vi "Vision.vi"() -> (3 "Done?":bool=TRUE)   [LabVIEW 2019]
uses:
  <vilib>/addons/control/pid/autopid.llb/PID autotuning parameters (adv).ctl
  <vilib>/Rock Robotics/WPI/Utilities/WPI_GetSetVariantRefNum.vi
  <vilib>/Rock Robotics/Network Tables/NT Write Boolean Array.vi
  <vilib>/Rock Robotics/Network Tables/NT Write Numeric Array.vi
  <vilib>/Rock Robotics/Network Tables/NT Read Boolean.vi
  <vilib>/Rock Robotics/Network Tables/NT Read Number.vi
  <vilib>/Rock Robotics/Network Tables/NT Write Boolean.vi
  <vilib>/addons/control/pid/NI_PID_autopid.lvlib
panel:
  out "tuning completed?":bool
  out "tuned PID gains":T1={"proportional gain (Kc)"=1.0, "integral time (Ti, min)"=0.01, "derivative time (Td, min)"=0.0} {"derivative time (Td, min)" format="%#.6g"; "integral time (Ti, min)" format="%#.6g"; "proportional gain (Kc)" format="%#.6g"}
  out "x/y":dbl
  in  "PID gains":T1={"proportional gain (Kc)"=0.07, "integral time (Ti, min)"=0.0033999999999999994, "derivative time (Td, min)"=0.05} {"derivative time (Td, min)" format="%.6f"; "integral time (Ti, min)" format="%.6f"; "proportional gain (Kc)" format="%.6f"}
  in  "On":bool
  out "Yaw":dbl
  out "Sample Slider 0":dbl(slide) scale=0.0..5.0
  out "Sample Boolean 1":bool
  out "Sample Boolean 0":bool
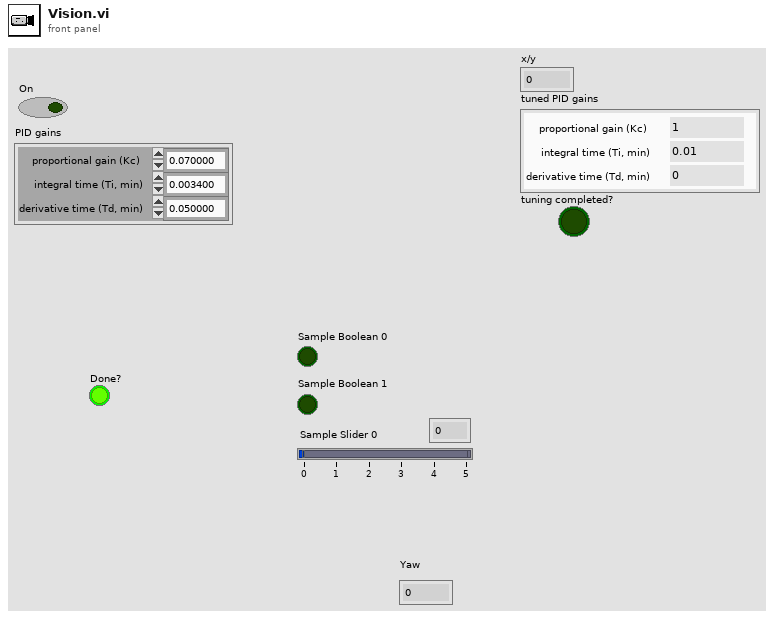
[diagram p1: front panel]
types:
  T1 = cluster{"proportional gain (Kc)":dbl, "integral time (Ti, min)":dbl, "derivative time (Td, min)":dbl}
  T2 = typedef "NI_PID_autopid.lvlib/PID autotuning parameters (adv).ctl" = cluster{"technique":u16, "type of controller":u16, "control specification":u16, "amplitude":dbl}
  T3 = typedef "WPI_EncoderDevRef.ctl" = cluster{"DevStatus":errorcluster, "EncoderIndex":T4, "CounterIndex":T5, "DistancePerCount":dbl, "Decoding Type":T6}
  T4 = typedef "FPGA_EncoderIdx.ctl" = enum8{"Enc 0", "Enc 1", "Enc 2", "Enc 3", "Enc 4", "Enc 5", "Enc 6", "Enc 7", "Invalid"}
  T5 = typedef "FPGA_CounterCtrSystemIndex.ctl" = enum8{"Ctr 0", "Ctr 1", "Ctr 2", "Ctr 3", "Ctr 4", "Ctr 5", "Ctr 6", "Ctr 7", "Invalid"}
  T6 = typedef "WPI_EncoderType.ctl" = enum16{"1x", "2x", "4x"}
  T7 = typedef "WPI_MotorControlDeviceRef.ctl" = cluster{"DeviceStatus":errorcluster, "Type":T8, "PWM":cluster{"PWM Channel":T9, "DeadBand":T10}, "CAN":cluster{"Device Number":u8, "SetOutput VI Ref":variant, "GetOutput VI Ref":variant, "Enable VI Ref":variant, "Disable VI Ref":variant, "Data":variant}, "Invert":bool, "DIO PWM":cluster{"PWM \"Enable\" Channel":T9, "DIOChannel":T11, "PWM Rate":dbl}}
  T8 = typedef "WPI_MotorControlType.ctl" = enum16{"PWM", "CAN", "DIO PWM"}
  T9 = typedef "FPGA_DIOPWMChannel.ctl" = enum8{"PWM 0", "PWM 1", "PWM 2", "PWM 3", "PWM 4", "PWM 5", "PWM 6", "PWM 7", "PWM 8", "PWM 9", "PWM MXP 0", "PWM MXP 1", "PWM MXP 2", "PWM MXP 3", "PWM MXP 4", "PWM MXP 5", "PWM MXP 6", "PWM MXP 7", "PWM MXP 8", "PWM MXP 9", "Invalid"}
  T10 = typedef "WPI_PWMDeadband.ctl" = cluster{"Name":string, "maxPositivePwm":i32, "minPositivePwm":i32, "centerPwm":i32, "maxNegativePwm":i32, "minNegativePwm":i32, "angularRange":u16}
  T11 = typedef "FPGA_DIOChannel.ctl" = enum8{"DIO 0", "DIO 1", "DIO 2", "DIO 3", "DIO 4", "DIO 5", "DIO 6", "DIO 7", "DIO 8", "DIO 9", "DIO MXP 0", "DIO MXP 1", "DIO MXP 2", "DIO MXP 3", "DIO MXP 4", "DIO MXP 5", "DIO MXP 6", "DIO MXP 7", "DIO MXP 8", "DIO MXP 9", "DIO MXP 10", "DIO MXP 11", "DIO MXP 12", "DIO MXP 13", "DIO MXP 14", "DIO MXP 15", "SPI Port CS1", "SPI Port CS2", "SPI Port CS3", "SPI Port MISO", "SPI Port MOSI", "Invalid"}
  T12 = typedef "WPI_JoystickDevRef.ctl" = cluster{"Device":T13}
  T13 = typedef "WPI_JoystickDeviceEnum.ctl" = enum16{"USB 0", "USB 1", "USB 2", "USB 3", "USB 4", "USB 5"}
  T14 = typedef "WPI_RobotDriveDevRef.ctl" = cluster{"DevStatus":errorcluster, "Motors[]":T7[], "Square Inputs":bool, "Max Output":dbl}
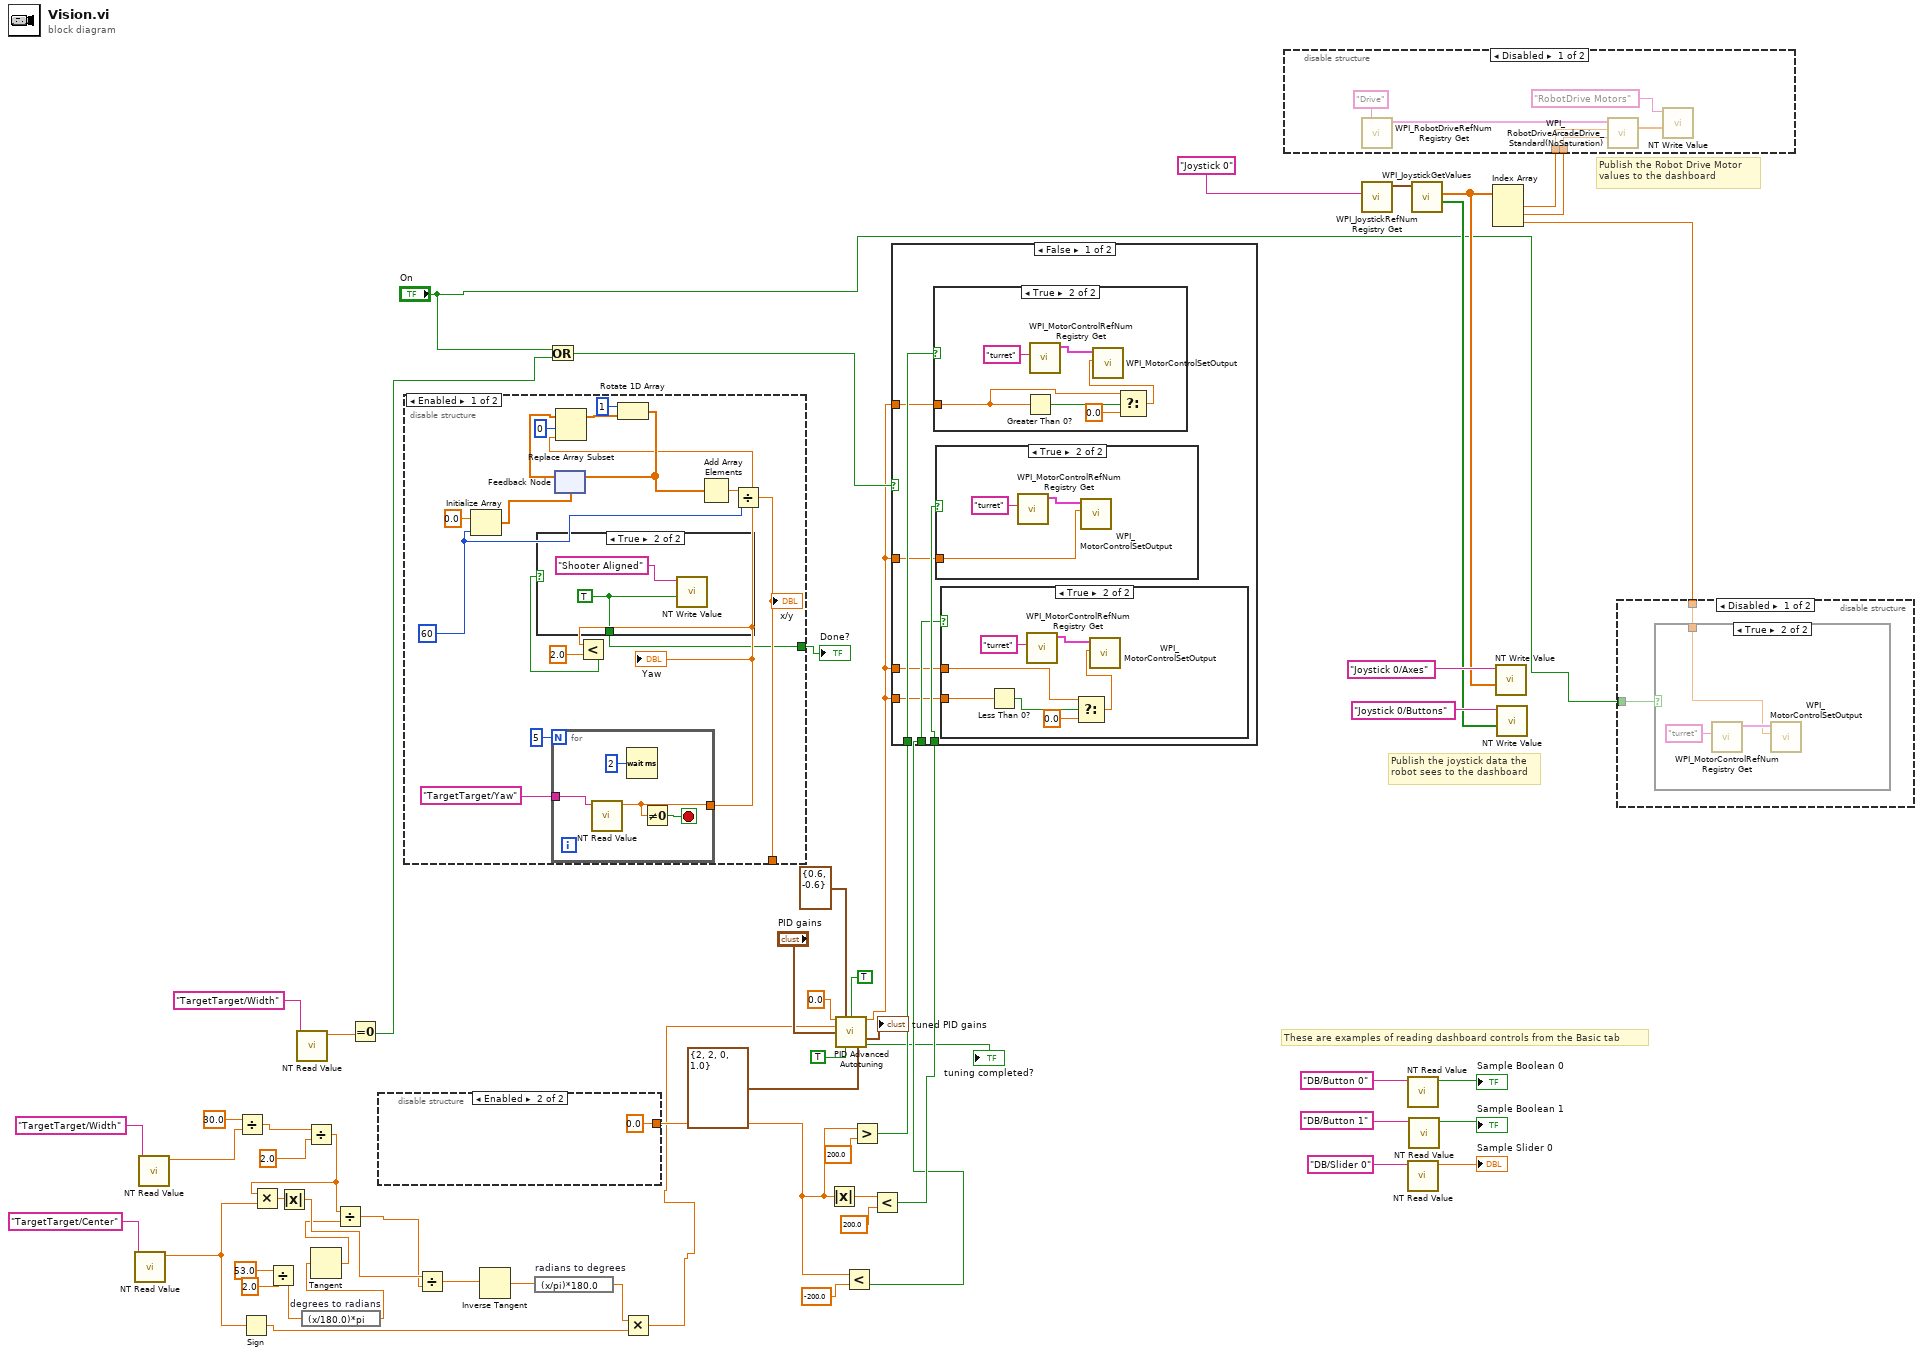
[diagram p0: block diagram]
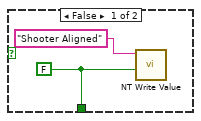
[diagram p2: hidden frame]
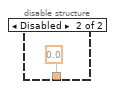
[diagram p3: hidden frame]
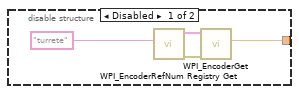
[diagram p4: hidden frame]
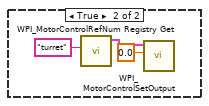
[diagram p11: hidden frame]
diagram:
  # "These are examples of reading dashboard controls from the Basic tab"
  # "Publish the Robot Drive Motor\nvalues to the dashboard"
  # "Publish the joystick data the\nrobot sees to the dashboard"
  n1 = call-poly <vilib>:"NT Read Value.vi"("Name"="TargetTarget/Center") -> ("Numeric"=w10:dbl)  [unwired: 9 in, 1 out]
  n2 = call-poly <vilib>:"NT Read Value.vi"("Name"="TargetTarget/Width") -> ("Numeric"=w20:dbl)  [unwired: 9 in, 1 out]
  n3 = Divide(x=30.0, y=w20) -> (x/y=w16:dbl)
  n4 = Sign(1:w10) -> (0:w8:dbl)
  n5 = Divide(x=53.0, y=2.0) -> (x/y=w7:dbl)
  n6 = call-poly <vilib>:"NT Read Value.vi"("Name"="TargetTarget/Width") -> ("Numeric"=w44:dbl)  [unwired: 9 in, 1 out]
  n7 = expression code="(x/180.0)*pi" "degrees to radians"(w7) -> (w6:dbl)
  n8 = Divide(x=w16, y=2.0) -> (x/y=w12:dbl)
  n9 = Multiply(x=w12, y=w10) -> (x*y=w15:dbl)
  n10 = Absolute Value(x=w15) -> (abs(x)=w14:dbl)
  n11 = Tangent(1:w6) -> (0:w5:dbl)
  n12 = Divide(x=w12, y=w5) -> (x/y=w4:dbl)
  n13 = Equal To 0?(x=w44) -> (x = 0?=w43:bool)
  n14 = disable-structure shown="Enabled" {
    disable-tunnel: [w60 0.0 ("Distance")] -> w35
    frame Disabled {
      n15 = call <vilib>:"WPI_EncoderRefNum Registry Get.vi"("refnum name"="turrete") -> ("error out"=w63:errorcluster, "EncoderDevRef"=w62:T3)  [unwired: 9 in]
      n16 = call <vilib>:"WPI_EncoderGet.vi"("error in (no error)"=w63, "EncoderDevRef"=w62) -> ("Distance"=w60:dbl)  [unwired: 4 in, 5 out]
    }
    frame Enabled {
    }
  }
  n17 = disable-structure shown="Enabled" {
    disable-tunnel: [w71 0.0] -> _
    disable-tunnel: [w65 _] -> w1
    frame Enabled {
      w72 = 60 ("dimension size")
      n18 = Initialize Array(0.0 ("element"), w72) -> (w75:dbl[])
      n19 = for {
        N: 5 -> [_]
        tunnel: [w87] -> w68
        tunnel: "TargetTarget/Yaw" ("Name") -> [w88]
        stop <- w85 stop-if-true
        n20 = call-poly <vilib>:"NT Read Value.vi"("Name"=w88) -> ("Numeric"=w87:dbl)  [unwired: 9 in, 1 out]
        n21 = Wait (ms)(milliseconds to wait=u32 2) -> ()  [unwired: 1 out]
        n22 = Not Equal To 0?(x=w87) -> (x != 0?=w85:bool)
      }
      "Yaw" <- w68
      n23 = feedback #1(w75) -> (w76:dbl[])
      n24 = Replace Array Subset(array=w76, new element=w68, index=0) -> (w78:dbl[])
      n25 = Less?(x=w68, y=2.0) -> (x < y?=w66:bool)
      n26 = case shown="True" w66 {
        tunnel: [w81 w83] -> w65
        frame False {
          w81 = FALSE ("Boolean")
          n27 = call-poly <vilib>:"NT Write Value.vi"("Boolean"=w81, "Name"="Shooter Aligned") -> ()  [unwired: 9 in, 1 out]
        }
        frame True {
          w83 = TRUE ("Boolean")
          n28 = call-poly <vilib>:"NT Write Value.vi"("Boolean"=w83, "Name"="Shooter Aligned") -> ()  [unwired: 9 in, 1 out]
        }
      }
      n29 = Rotate 1D Array(1:w78, 2:1 ("n")) -> (0:w74:dbl[])
      n30 = feedback-in #1(w74) -> ()
      n31 = Add Array Elements(numeric array=w74) -> (sum=w73:dbl)
      n32 = Divide(x=w73, y=w72) -> (x/y=w71:dbl)
      "x/y" <- w71
    }
    frame Disabled {
    }
  }
  "Done?" <- w1
  n33 = Divide(x=w14, y=w4) -> (x/y=w13:dbl)
  n34 = Inverse Tangent(1:w13) -> (0:w11:dbl)
  n35 = expression code="(x/pi)*180.0" "radians to degrees"(w11) -> (w9:dbl)
  n36 = Or(x="On", y=w43) -> (x .or. y?=w34:bool)
  n37 = Multiply(x=w9, y=w8) -> (x*y=w2:dbl)
  n38 = Absolute Value(x=w35) -> (abs(x)=w42:dbl)
  n39 = call <vilib>:"PID Advanced Autotuning.vi"("setpoint"=0.0, "output range"=cluster{"output high":dbl, "output low":dbl} {"output high"=0.6, "output low"=-0.6}, "auto? (F)"=TRUE ("auto? (T)"), "process variable"=w2, "PID gains"="PID gains", "reinitialize? (F)"=TRUE, "autotuning parameters"=T2 {"technique"=2, "type of controller"=2, "control specification"=0, "amplitude"=1.0}) -> ("output"=w33:dbl, "tuned PID gains"=→"tuned PID gains":T1, "tuning completed?"=→"tuning completed?":bool)  [unwired: 6 in]
  n40 = Less?(x=w35, y=-200.0) -> (x < y?=w38:bool)
  n41 = Greater?(x=w35, y=200.0) -> (0:w36:bool)
  n42 = Less?(x=w42, y=200.0) -> (x < y?=w40:bool)
  n43 = case shown="False" w34 {
    tunnel: w40 -> [w96 _]
    tunnel: w38 -> [w95 _]
    tunnel: w36 -> [w94 _]
    tunnel: w33 -> [w93 _]
    tunnel: w33 -> [w92 _]
    tunnel: w33 -> [w91 _]
    tunnel: w33 -> [w90 _]
    frame False {
      n44 = case shown="True" w94 {
        tunnel: w91 -> [_ w107]
        frame False {
        }
        frame True {
          n45 = Greater Than 0?(x=w107) -> (x > 0?=w111:bool)
          n46 = call <vilib>:"WPI_MotorControlRefNum Registry Get.vi"("refnum name"="turret") -> ("MotorControlDevRef"=w112:T7)  [unwired: 9 in, 1 out]
          n47 = Select(t=w107, s=w111, f=0.0) -> (s? t:f=w109:dbl)
          n48 = call <vilib>:"WPI_MotorControlSetOutput.vi"("Output"=w109, "MotorControlDevRef"=w112) -> ()  [unwired: 7 in, 3 out]
        }
      }
      n49 = case shown="True" w96 {
        tunnel: w93 -> [_ w104]
        frame False {
        }
        frame True {
          n50 = call <vilib>:"WPI_MotorControlRefNum Registry Get.vi"("refnum name"="turret") -> ("MotorControlDevRef"=w106:T7)  [unwired: 9 in, 1 out]
          n51 = call <vilib>:"WPI_MotorControlSetOutput.vi"("Output"=w104, "MotorControlDevRef"=w106) -> ()  [unwired: 7 in, 3 out]
        }
      }
      n52 = case shown="True" w95 {
        tunnel: w92 -> [_ w98]
        tunnel: w90 -> [_ w97]
        frame False {
        }
        frame True {
          n53 = Less Than 0?(x=w97) -> (x < 0?=w101:bool)
          n54 = call <vilib>:"WPI_MotorControlRefNum Registry Get.vi"("refnum name"="turret") -> ("MotorControlDevRef"=w103:T7)  [unwired: 9 in, 1 out]
          n55 = Select(t=w98, s=w101, f=0.0) -> (s? t:f=w99:dbl)
          n56 = call <vilib>:"WPI_MotorControlSetOutput.vi"("Output"=w99, "MotorControlDevRef"=w103) -> ()  [unwired: 7 in, 3 out]
        }
      }
    }
    frame True {
      n57 = call <vilib>:"WPI_MotorControlRefNum Registry Get.vi"("refnum name"="turret") -> ("MotorControlDevRef"=w115:T7)  [unwired: 9 in, 1 out]
      n58 = call <vilib>:"WPI_MotorControlSetOutput.vi"("Output"=0.0, "MotorControlDevRef"=w115) -> ()  [unwired: 7 in, 3 out]
    }
  }
  n59 = call <vilib>:"WPI_JoystickRefNum Registry Get.vi"("refnum name"="Joystick 0") -> ("JoystickDevRef"=w57:T12)  [unwired: 1 in, 9 out]
  n60 = call-poly <vilib>:"NT Read Value.vi"("Name"="DB/Button 0" ("refnum name")) -> ("Boolean"=→"Sample Boolean 0":bool)  [unwired: 9 in, 1 out]
  n61 = call-poly <vilib>:"NT Read Value.vi"("Name"="DB/Slider 0" ("refnum name")) -> ("Numeric"=→"Sample Slider 0":dbl)  [unwired: 9 in, 1 out]
  n62 = call-poly <vilib>:"NT Read Value.vi"("Name"="DB/Button 1" ("refnum name")) -> ("Boolean"=→"Sample Boolean 1":bool)  [unwired: 9 in, 1 out]
  n63 = call <vilib>:"WPI_JoystickGetValues.vi"("JoystickDevRef"=w57) -> ("Buttons"=w52:bool[], "Axes"=w53:dbl[])  [unwired: 6 in, 3 out]
  n64 = Index Array(array=w53) -> (element #1=w59:dbl, element #2=w56:dbl, element #3=w24:dbl)  [unwired: 3 in]
  n65 = disable-structure shown="Disabled" {
    disable-tunnel: w59 -> [w119 _]
    disable-tunnel: w56 -> [w118 _]
    frame Disabled {
      n66 = call <vilib>:"WPI_RobotDriveRefNum Registry Get.vi"("refnum name"="Drive") -> ("RobotDriveDevRef"=w120:T14)  [unwired: 1 in, 9 out]
      n67 = call <vilib>:"WPI_RobotDriveArcadeDrive_Standard(NoSaturation).vi"("Y axis value"=w118, "X axis value"=w119, "RobotDriveDevRef"=w120) -> ("Motor Values"=w117:dbl[])  [unwired: 1 in, 7 out]
      n68 = call-poly <vilib>:"NT Write Value.vi"("Numeric Array"=w117, "Name"="RobotDrive Motors") -> ()  [unwired: 9 in, 1 out]
    }
    frame Enabled {
    }
  }
  n69 = call-poly <vilib>:"NT Write Value.vi"("Numeric Array"=w53, "Name"="Joystick 0/Axes") -> ()  [unwired: 9 in, 1 out]
  n70 = call-poly <vilib>:"NT Write Value.vi"("Boolean Array"=w52, "Name"="Joystick 0/Buttons") -> ()  [unwired: 9 in, 1 out]
  n71 = disable-structure shown="Disabled" {
    disable-tunnel: "On" -> [w123 _]
    disable-tunnel: w24 -> [w122 _]
    frame Disabled {
      n72 = case shown="True" w123 {
        tunnel: w122 -> [_ w124]
        frame False {
        }
        frame True {
          n73 = call <vilib>:"WPI_MotorControlRefNum Registry Get.vi"("refnum name"="turret") -> ("MotorControlDevRef"=w126:T7)  [unwired: 9 in, 1 out]
          n74 = call <vilib>:"WPI_MotorControlSetOutput.vi"("Output"=w124, "MotorControlDevRef"=w126) -> ()  [unwired: 7 in, 3 out]
        }
      }
    }
    frame Enabled {
    }
  }
